vi "start_acquisition.vi"(9 "Input\nparameters":T2={"Frame rate (ms)"=2000, "Worm Strain"="N2", "Time t"=0, "State"=enum."Image acquisition", "Acquisition time"=0.0, "Maximum # of images"=100000, "#TTL"=0, "time of third ttl "=100000, "ImSub Value"=0, "Time of last TTL"=0, "# Rows"=2, "# Columns"=2, "number of adjacentTTL"=0, "Sleep Deprivation status"="", "Sleep Detection"=FALSE, "Time of first sleep detection"=0, "# Sleep detections"=0, "Time max # adjacent TTL"=-10000, "Image t-1"=[], "Image t"=[]} {"# Columns" items=["1"=1, "2"=2, "3"=3, "4"=4]; "# Rows" items=["1"=1, "2"=2, "3"=3, "4"=4]}, 10 "Frame rate":u32=2000) -> (1 "Output\nparameters":T2={"Frame rate (ms)"=2000, "Worm Strain"="N2", "Time t"=0, "State"=enum."Image acquisition", "Acquisition time"=0.0, "Maximum # of images"=100000, "#TTL"=0, "time of third ttl "=100000, "ImSub Value"=0, "Time of last TTL"=0, "# Rows"=2, "# Columns"=2, "number of adjacentTTL"=0, "Sleep Deprivation status"="", "Sleep Detection"=FALSE, "Time of first sleep detection"=0, "# Sleep detections"=0, "Time max # adjacent TTL"=-10000, "Image t-1"=[], "Image t"=[]} {"# Columns" items=["1"=1, "2"=2, "3"=3, "4"=4]; "# Rows" items=["1"=1, "2"=2, "3"=3, "4"=4]}, 2 "Acquisition\nsuccessfull":bool)   [LabVIEW 2011]
uses:
  state.ctl
panel:
  out "?":u32
  # "General settings"
  # "Select number of animals"
  # "Row"
  # "Column"
  # "General settings"
  # "Select number of animals"
  # "Row"
  # "Column"
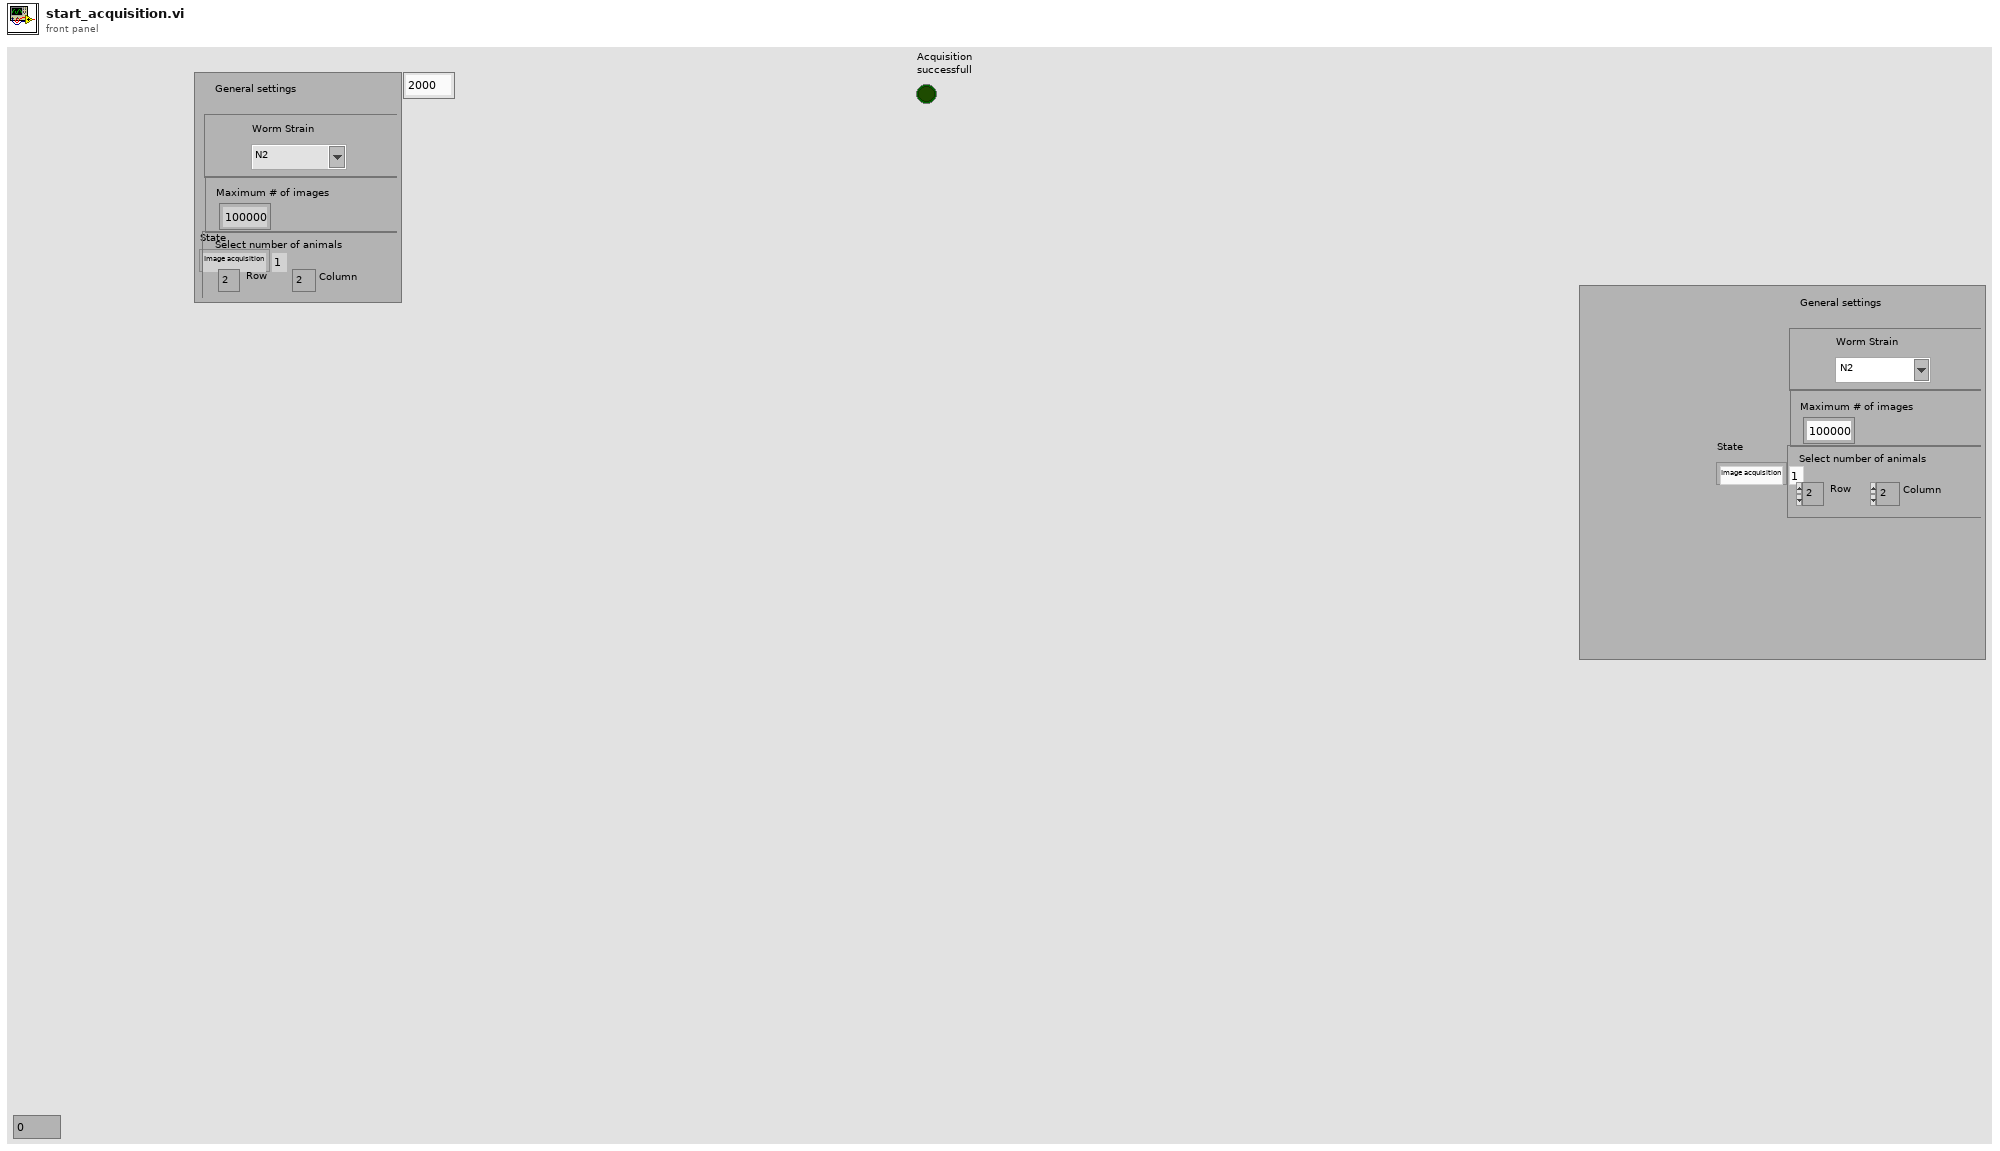
[diagram p1: front panel]
types:
  T1 = typedef "state.ctl" = enum16{"Initialize measurement", "Image acquisition", "Image processing", "Sleep detection", "Control TTL protocol ", "Sleep deprivation", "Update image & exit condition", "Wait "}
  T2 = cluster{"Frame rate (ms)":u32, "Worm Strain":string, "Time t":i32, "State":T1, "Acquisition time":dbl, "Maximum # of images":i32, "#TTL":i32, "time of third ttl ":i32, "ImSub Value":i32, "Time of last TTL":i32, "# Rows":u32, "# Columns":u32, "number of adjacentTTL":i32, "Sleep Deprivation status":string, "Sleep Detection":bool, "Time of first sleep detection":i32, "# Sleep detections":i32, "Time max # adjacent TTL":i32, "Image t-1":i32[][], "Image t":i32[][]}
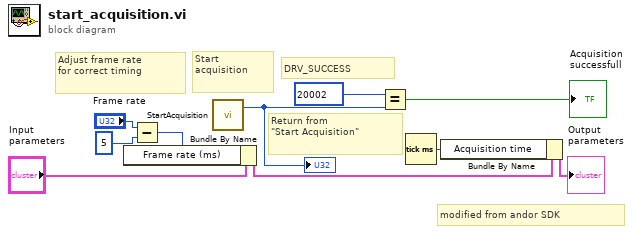
[diagram p0: block diagram]
diagram:
  # "Adjust frame rate\nfor correct timing"
  # "modified from andor SDK"
  # "Start\nacquisition"
  # "DRV_SUCCESS"
  # "Return from\n\"Start Acquisition\""
  n1 = Subtract(x="Frame rate", y=u32 5 ("Frame rate (ms)")) -> (x-y=w1:u32)
  n2 = Bundle By Name(cluster="Input\nparameters", "Frame rate (ms)"=w1) -> (w5:T2)
  n3 = call <userlib>:"StartAcquisition.vi"() -> ("DLL error code"=w10:u32)  [unwired: 2 in, 1 out]
  "?" <- w10
  n4 = Equal?(x=20002, y=w10) -> (x = y?=→"Acquisition\nsuccessfull":bool)
  n5 = Tick Count (ms)() -> (millisecond timer value=w8:u32)
  n6 = Bundle By Name(cluster=w5, "Acquisition time"=w8) -> (→"Output\nparameters":T2)
